vi "Array_2_Xml.vi"() -> ()   [LabVIEW 2023]
uses:
  TypeDef/Method_Info.ctl
panel:
  out "xml string":string
  in  "Type_Fits":T1[](array[typedef])
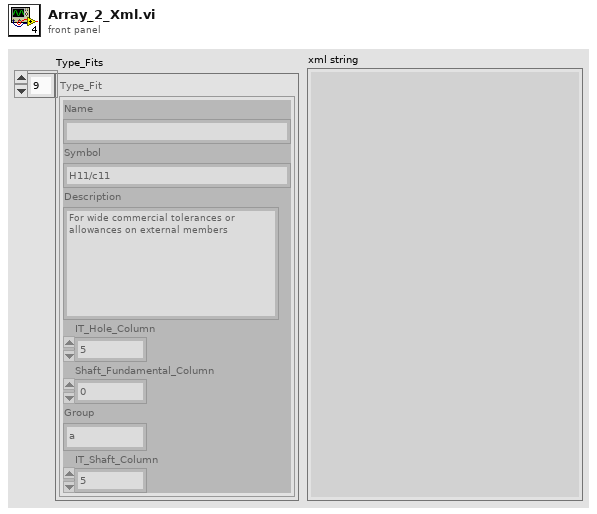
[diagram p1: front panel]
types:
  T1 = typedef "Method_Info.ctl" = cluster{"Name":string, "Symbol":string, "Description":string, "IT_Hole_Column":i32, "Shaft_Fundamental_Column":i32, "Group":string, "IT_Shaft_Column":i32}
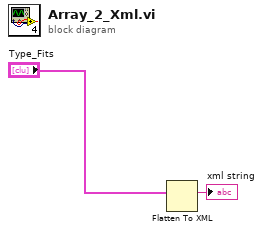
[diagram p0: block diagram]
diagram:
  n1 = Flatten To XML(6:"Type_Fits") -> (2:→"xml string":string)
